vi "readFromXML.vi"(8 "error in (no error)":errorcluster, 10 "XML in":string="<MccDebug>\n  <debugLevel>1</debugLevel>\n</MccDebug>", 11 "MccDebug in":refnum<class "MccDebug.lvclass">) -> (0 "error out":errorcluster, 3 "MccDebug out":refnum<class "MccDebug.lvclass">)   [LabVIEW 2014, in "TCSDataDefinitions.lvlib" / "TCSMountControlCommand.lvlib" / "CommandsForAllAxes.lvlib" / "MccDebug.lvclass"]
uses:
  MccDebug.lvclass
  TCSCommand/Enumerations/TCSDebuLevelTypes.ctl
  MccDebug.lvclass/MccDebug.ctl
  CommandsForAllAxes.lvclass
  <userlib>/Common/XML/XMLParser/XMLParser.lvclass
  TCSCommand/TCSCommand.lvlib
panel:
  out "debugLevel":T1=enum."1"
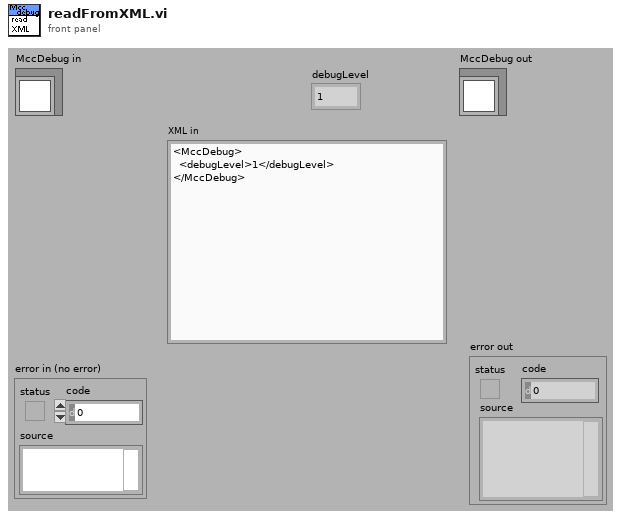
[diagram p1: front panel]
types:
  T1 = typedef "TCSDataDefinitions.lvlib/TCSCommand.lvlib/TCSDebuLevelTypes.ctl" = enum16{"0", "1", "2", "3", "4", "5", "6", "7", "8", "9", "10"}
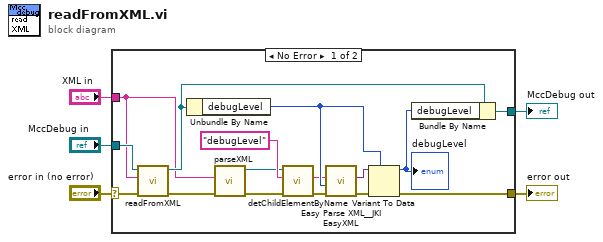
[diagram p0: block diagram]
diagram:
  n1 = case shown="No Error" "error in (no error)" {
    selector: "error in (no error)" -> [w8 w23]
    tunnel: [w18 w23] -> w4
    tunnel: [w21 w22] -> w2
    tunnel: "MccDebug in" -> [w11 w22]
    tunnel: "XML in" -> [w9 _]
    frame No Error {
      n2 = call-parent "readFromXML.vi"("error in (no error)"=w8, "XML in"=w9, "CommandsForAllAxes in"=w11) -> ("error out"=w7:errorcluster, "CommandsForAllAxes out"=w10:refnum<class "MccDebug.lvclass">)  [unwired: 7 in]
      n3 = Unbundle By Name(w10) -> ("debugLevel"=w16:T1)
      n4 = call <userlib>:"parseXML.vi"("error in (no error)"=w7, "XMLString in"=w9) -> ("error out"=w15:errorcluster, "Element out"=w6:refnum<class "XMLParser.lvclass">)  [unwired: 8 in]
      n5 = call <userlib>:"detChildElementByName.vi"("error in (no error)"=w15, "childName"="debugLevel" ("ChildName"), "Element in"=w6) -> ("error out"=w14:errorcluster, "childXML"=w12:string)  [unwired: 5 in, 2 out]
      n6 = call <vilib>:"Easy Parse XML__JKI EasyXML.vi"("error in (no error)"=w14, "LabVIEW Data (Type)"=w16, "XML String"=w12) -> ("error out"=w19:errorcluster, "LabVIEW Data"=w20:variant)  [unwired: 7 in]
      n7 = Variant To Data(error in=w19, type=w16, Variant=w20) -> (data=w17:T1, error out=w18:errorcluster)
      "debugLevel" <- w17
      n8 = Bundle By Name(cluster=w10, "debugLevel"=w17) -> (w21:refnum<class "MccDebug.lvclass">)
    }
    frame Error {
    }
  }
  "error out" <- w4
  "MccDebug out" <- w2
